vi "cold_cathode_control.vi"(11 "Cold Cathode Gauge Channel":tag="Dev3/ai6") -> (3 "Cold Cathode Gauge Pressure":dbl)   [LabVIEW 2014]
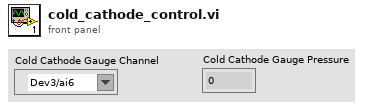
[diagram p1: front panel]
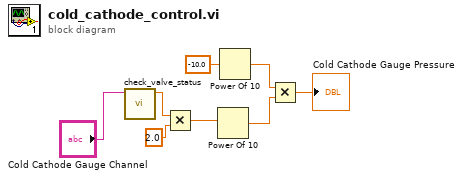
[diagram p0: block diagram]
diagram:
  n1 = call "check_valve_status.vi"("Channel 1"="Cold Cathode Gauge Channel") -> ("Ch. 1 value"=w4:dbl)  [unwired: 10 in]
  n2 = Multiply(x=w4, y=2.0) -> (x*y=w2:dbl)
  n3 = Power Of 10(x=w2) -> (10^x=w5:dbl)
  n4 = Power Of 10(x=-10.0) -> (10^x=w6:dbl)
  n5 = Multiply(x=w6, y=w5) -> (x*y=→"Cold Cathode Gauge Pressure":dbl)
